vi "Get Output Values.vi"(6 "Initialize Indices":cluster{"Index Bool":bool, "Indices":i32[]}, 7 "Step GUIDs":string[](array[string]), 8 "error in (no error)":errorcluster, 9 "Channel Type Array":string[](array[string]), 10 "Step Results":T1(array[cluster]), 11 "Step GUID Array":string[](array[string])) -> (0 "error out":errorcluster, 3 "Output Values":dbl[](array[numeric]))   [LabVIEW 2012, in "Shared Variable Custom Device.lvlib"]
uses:
  Shared Variable Custom Device.lvlib
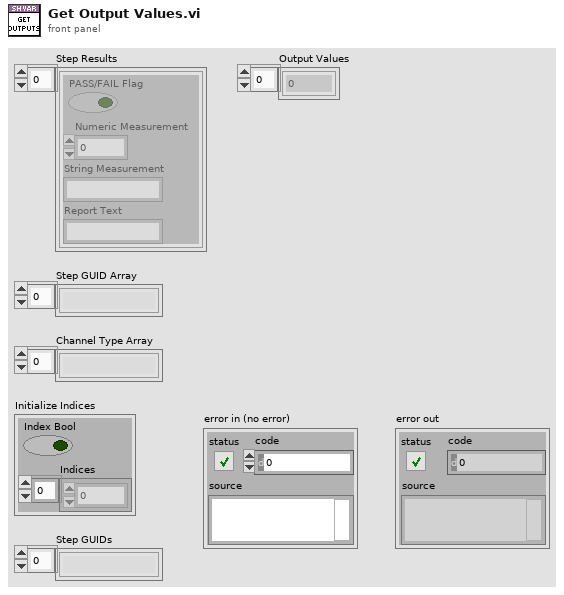
[diagram p1: front panel]
types:
  T1 = cluster{"PASS/FAIL Flag":bool, "Numeric Measurement":dbl, "String Measurement":string, "Report Text":string}[]
  T2 = cluster{"PASS/FAIL Flag":bool, "Numeric Measurement":dbl, "String Measurement":string, "Report Text":string}
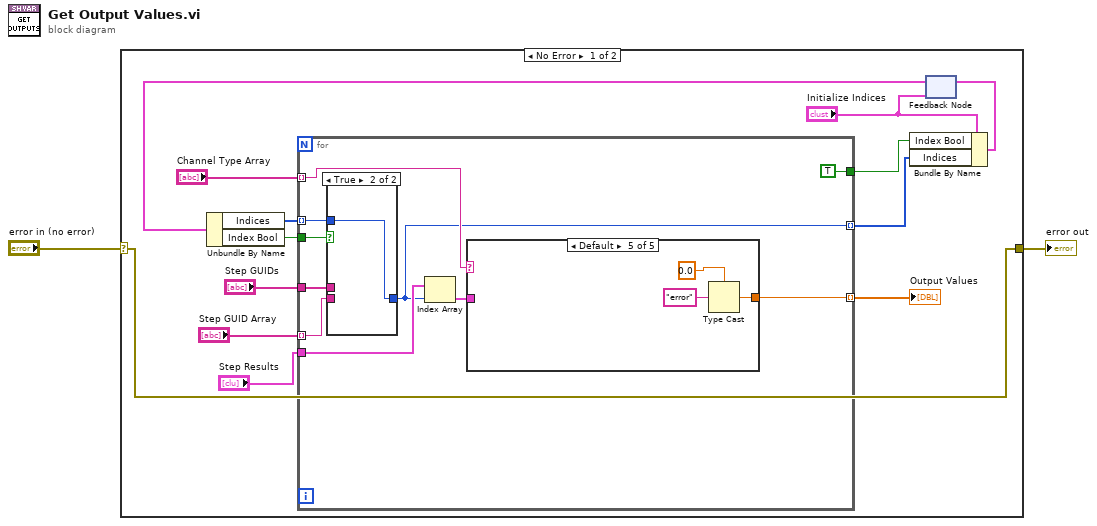
[diagram p0: block diagram]
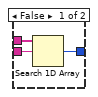
[diagram p2: hidden frame]
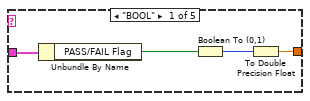
[diagram p3: hidden frame]
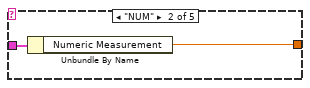
[diagram p4: hidden frame]
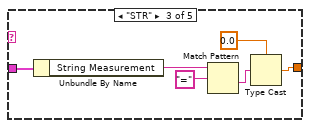
[diagram p5: hidden frame]
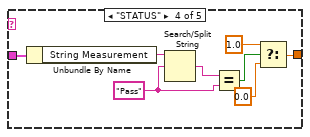
[diagram p6: hidden frame]
diagram:
  n1 = case shown="No Error" "error in (no error)" {
    selector: "error in (no error)" -> [w3 w53]
    tunnel: [w3 w53] -> w1
    frame No Error {
      n2 = feedback #1("Initialize Indices") -> (w10:cluster{"Index Bool":bool, "Indices":i32[]})
      n3 = Unbundle By Name(w10) -> ("Indices"=w12:i32[], "Index Bool"=w11:bool)
      n4 = for {
        tunnel: "Step GUIDs" -> [w25]
        tunnel: "Step GUID Array" -> [w16] mode=indexing
        tunnel: "Step Results" -> [w24]
        tunnel: "Channel Type Array" -> [w23] mode=indexing
        tunnel: [w17] -> w15 mode=indexing
        tunnel: [w18] -> w14 mode=indexing
        tunnel: [TRUE] -> w9
        tunnel: w11 -> [w20]
        tunnel: w12 -> [w19] mode=indexing
        n5 = case shown="True" w20 {
          tunnel: w25 -> [w28 _]
          tunnel: w16 -> [w27 _]
          tunnel: [w26 w29] -> w18
          tunnel: w19 -> [_ w29]
          frame False {
            n6 = Search 1D Array(1D array=w28, element=w27) -> (index of element=w26:i32)  [unwired: 1 in]
          }
          frame True {
          }
        }
        n7 = Index Array(array=w24, index=w18) -> (element=w22:T2)
        n8 = case shown="Default" w23 {
          tunnel: w22 -> [w33 w35 w41 w49 _]
          tunnel: [w30 w34 w36 w45 w52] -> w17
          frame "BOOL" {
            n9 = Unbundle By Name(w33) -> ("PASS/FAIL Flag"=w32:bool)
            n10 = Boolean To (0,1)(Boolean=w32) -> (0, 1=w31:i16)
            n11 = To Double Precision Float(number=w31) -> (double precision float=w30:dbl)
          }
          frame "NUM" {
            n12 = Unbundle By Name(w35) -> ("Numeric Measurement"=w34:dbl)
          }
          frame "STR" {
            n13 = Unbundle By Name(w41) -> ("String Measurement"=w40:string)
            n14 = Match Pattern(string=w40, regular expression="=") -> (after substring=w37:string)  [unwired: 1 in, 3 out]
            n15 = Type Cast(type=0.0, x=w37) -> (*(type *) &x=w36:dbl)
          }
          frame "STATUS" {
            w46 = "Pass" ("regular expression")
            n16 = Unbundle By Name(w49) -> ("String Measurement"=w48:string)
            n17 = Search/Split String(string=w48, search string/char (-)=w46) -> (match + rest of string=w47:string)  [unwired: 1 in, 2 out]
            n18 = Equal?(x=w47, y=w46) -> (x = y?=w44:bool)
            n19 = Select(t=1.0, s=w44, f=0.0) -> (s? t:f=w45:dbl)
          }
          frame Default {
            n20 = Type Cast(type=0.0, x="error") -> (*(type *) &x=w52:dbl)
          }
        }
      }
      "Output Values" <- w15
      n21 = Bundle By Name(cluster="Initialize Indices", "Index Bool"=w9, "Indices"=w14) -> (w8:cluster{"Index Bool":bool, "Indices":i32[]})
      n22 = feedback-in #1(w8) -> ()
    }
    frame Error {
    }
  }
  "error out" <- w1
